vi "Logarithm Fit (LS).vi"(0 "Y":dbl[](array[numeric]), 5 "X":dbl[](array[numeric]), 7 "Weight":dbl[](array[numeric]), 9 "base of logarithm":dbl(ring)=2.71828 items=["e"=2.71828, "2"=2.0, "10"=10.0]) -> (4 "Best Logarithm Fit":dbl[](array[numeric]), 6 "amplitude":dbl, 8 "scale":dbl, 14 "residue":dbl, 15 "error":i32)   [LabVIEW 2014, in "NI_AALPro.lvlib"]
uses:
  NI_AALPro.lvlib
  lvanlys.dll
panel:
  # "LS Logarithm Fit"
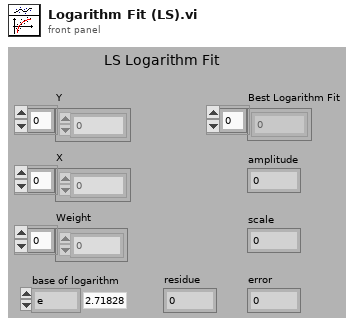
[diagram p1: front panel]
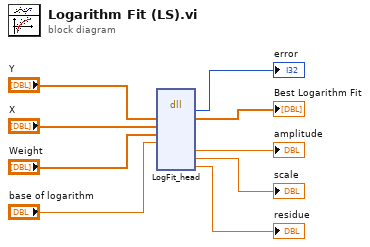
[diagram p0: block diagram]
diagram:
  n1 = dll-call lib="C:/Program Files (x86)/National Instruments/LabVIEW 2014/resource/lvanlys.*" fn="LogFit_head"("yH"="Y", "xH"="X", "weight"="Weight", "base"="base of logarithm") -> (→"error":i32, "yH"=→"Best Logarithm Fit":dbl[], "amplitude"=→"amplitude":dbl, "scale"=→"scale":dbl, "mse"=→"residue":dbl)  [unwired: 9 in, 2 out]
